vi "Start All DDS Communication Actors.vi"(8 "error in":errorcluster, 11 "SCADA in":refnum<class "EMS.lvclass">) -> (0 "error out":errorcluster, 3 "SCADA out":refnum<class "EMS.lvclass">)   [LabVIEW 2018, in "EMS Core.lvlib" / "EMS.lvclass"]
uses:
  EMS.lvclass
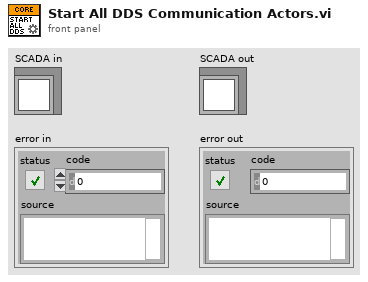
[diagram p1: front panel]
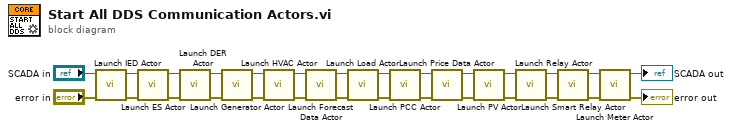
[diagram p0: block diagram]
diagram:
  n1 = call "Launch IED Actor.vi"("error in"="error in", "SCADA in"="SCADA in") -> ("error out"=w3:errorcluster, "SCADA out"=w2:refnum<class "EMS.lvclass">)  [unwired: 8 in]
  n2 = call "Launch ES Actor.vi"("error in"=w3, "SCADA in"=w2) -> ("error out"=w4:errorcluster, "SCADA out"=w5:refnum<class "EMS.lvclass">)  [unwired: 8 in]
  n3 = call "Launch DER Actor.vi"("error in"=w4, "SCADA in"=w5) -> ("error out"=w27:errorcluster, "SCADA out"=w26:refnum<class "EMS.lvclass">)  [unwired: 8 in]
  n4 = call "Launch Generator Actor.vi"("error in"=w27, "SCADA in"=w26) -> ("error out"=w28:errorcluster, "SCADA out"=w25:refnum<class "EMS.lvclass">)  [unwired: 8 in]
  n5 = call "Launch HVAC Actor.vi"("error in"=w28, "SCADA in"=w25) -> ("error out"=w6:errorcluster, "SCADA out"=w7:refnum<class "EMS.lvclass">)  [unwired: 8 in]
  n6 = call "Launch Forecast Data Actor.vi"("error in"=w6, "SCADA in"=w7) -> ("error out"=w9:errorcluster, "SCADA out"=w8:refnum<class "EMS.lvclass">)  [unwired: 8 in]
  n7 = call "Launch Load Actor.vi"("error in"=w9, "SCADA in"=w8) -> ("error out"=w10:errorcluster, "SCADA out"=w11:refnum<class "EMS.lvclass">)  [unwired: 8 in]
  n8 = call "Launch PCC Actor.vi"("error in"=w10, "SCADA in"=w11) -> ("error out"=w13:errorcluster, "SCADA out"=w12:refnum<class "EMS.lvclass">)  [unwired: 8 in]
  n9 = call "Launch Price Data Actor.vi"("error in"=w13, "SCADA in"=w12) -> ("error out"=w14:errorcluster, "SCADA out"=w15:refnum<class "EMS.lvclass">)  [unwired: 8 in]
  n10 = call "Launch PV Actor.vi"("error in"=w14, "SCADA in"=w15) -> ("error out"=w17:errorcluster, "SCADA out"=w16:refnum<class "EMS.lvclass">)  [unwired: 8 in]
  n11 = call "Launch Relay Actor.vi"("error in"=w17, "SCADA in"=w16) -> ("error out"=w18:errorcluster, "SCADA out"=w19:refnum<class "EMS.lvclass">)  [unwired: 8 in]
  n12 = call "Launch Smart Relay Actor.vi"("error in"=w18, "SCADA in"=w19) -> ("error out"=w21:errorcluster, "SCADA out"=w20:refnum<class "EMS.lvclass">)  [unwired: 8 in]
  n13 = call "Launch Meter Actor.vi"("error in"=w21, "SCADA in"=w20) -> ("error out"=→"error out":errorcluster, "SCADA out"=→"SCADA out":refnum<class "EMS.lvclass">)  [unwired: 8 in]
